vi "Store Waveform to Ref Channel.vi"(8 "error in (no error)":errorcluster, 9 "Reference (8:Reference1)":u16(ring)=8 items=["Reference 1"=8, "Reference 2"=9, "Reference 3"=10, "Reference 4"=11], 10 "Source (0: Channel 1)":u16(ring) items=["Channel 1", "Channel 2", "Channel 3", "Channel 4", "Math 1", "Math 2", "Math 3", "Math 4", "Reference 1", "Reference 2", "Reference 3", "Reference 4"], 11 "VISA resource name":refnum<visa-resource-name>) -> (0 "error out":errorcluster, 3 "VISA resource name out":refnum<visa-resource-name>)   [LabVIEW 2011, in "Tektronix 7000 Series.lvlib"]
doc: "Stores a waveform to a reference channel."
uses:
  Tektronix 7000 Series.lvlib
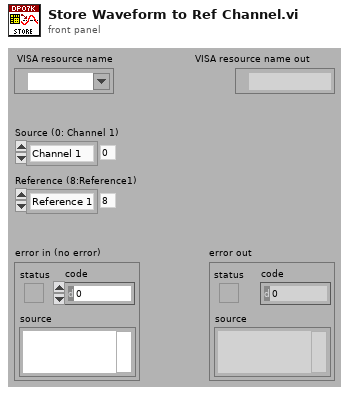
[diagram p1: front panel]
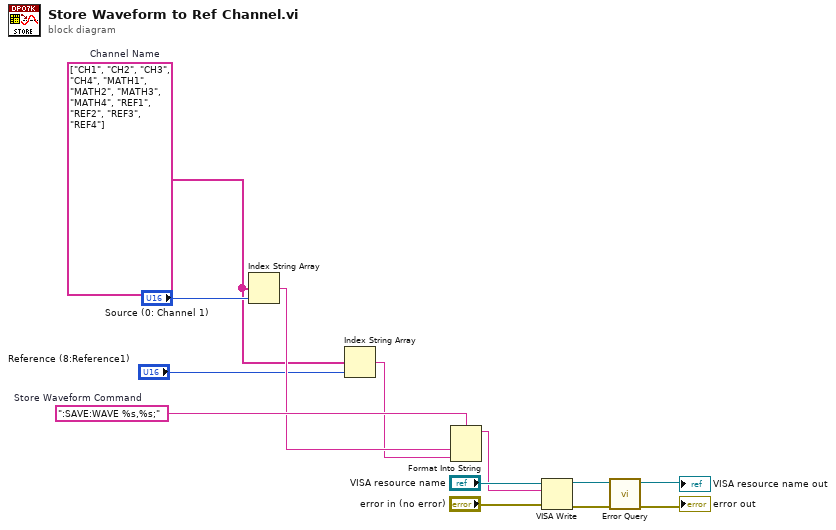
[diagram p0: block diagram]
diagram:
  w6 = string[] ["CH1", "CH2", "CH3", "CH4", "MATH1", "MATH2", "MATH3", "MATH4", "REF1", "REF2", "REF3", "REF4"]  # Channel Name
  w12 = ":SAVE:WAVE %s,%s;"  # Store Waveform Command
  n1 = Index String Array(1:"Source (0: Channel 1)", 2:w6) -> (0:w11:string)  [unwired: 1 in]
  n2 = Index String Array(1:"Reference (8:Reference1)", 2:w6) -> (0:w10:string)  [unwired: 1 in]
  n3 = Format Into String(format string=w12, w11, w10) -> (resulting string=w7:string)  [unwired: 2 in, 1 out]
  n4 = VISA Write(VISA resource name="VISA resource name", write buffer=w7, error in (no error)="error in (no error)") -> (VISA resource name out=w4:refnum<visa-resource-name>, error out=w3:errorcluster)  [unwired: 1 out]
  n5 = call "Error Query.vi"("error in (no error)"=w3, "VISA resource name"=w4) -> ("error out"=→"error out":errorcluster, "VISA resource name out"=→"VISA resource name out":refnum<visa-resource-name>)  [unwired: 6 in, 2 out]
